vi "create tiff file path.vi"(8 "error in (no error)":errorcluster, 9 "dcimg name":string, 10 "cxd folder Path":path) -> (0 "error IO":errorcluster, 2 "tiff file path":path, 3 "tiff folder path":path)   [LabVIEW 2012, in "DAQOrcaFlash.lvclass"]
uses:
  DAQOrcaFlash.lvclass
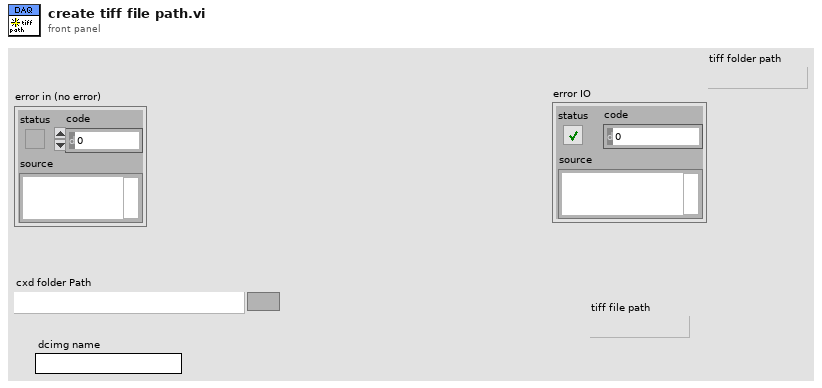
[diagram p1: front panel]
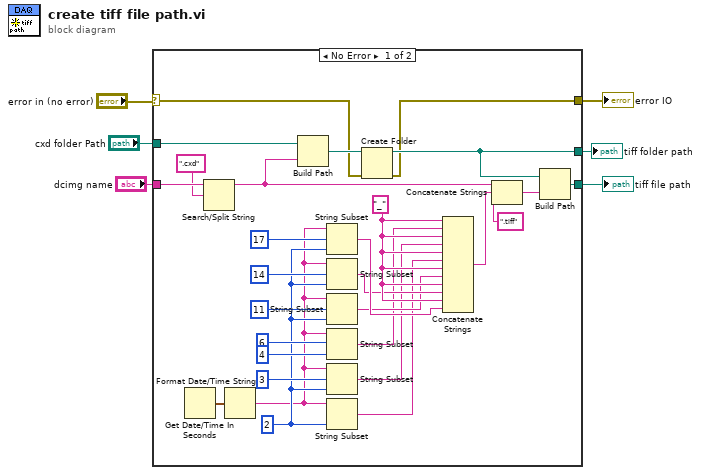
[diagram p0: block diagram]
diagram:
  n1 = case shown="No Error" "error in (no error)" {
    selector: "error in (no error)" -> [w8 w35]
    tunnel: "dcimg name" -> [w16 _]
    tunnel: [w7 w35] -> w4
    tunnel: [w11 _] -> w3
    tunnel: "cxd folder Path" -> [w10 _]
    tunnel: [w9 _] -> w1
    frame No Error {
      w34 = "_" ("string")
      w21 = 2 ("length (rest)")
      n2 = Get Date/Time In Seconds() -> (seconds since 1Jan1904=w19:timestamp)
      n3 = Search/Split String(string=w16, search string/char (-)=".cxd") -> (substring before match=w13:string)  [unwired: 1 in, 2 out]
      n4 = Format Date/Time String(seconds (now)=w19) -> (date/time string=w20:string)  [unwired: 2 in]
      n5 = Build Path(base path=w10, name or relative path=w13) -> (appended path=w14:path)
      n6 = String Subset(string=w20, offset (0)=17, length (rest)=w21) -> (substring=w33:string)
      n7 = String Subset(string=w20, offset (0)=14, length (rest)=w21) -> (substring=w32:string)
      n8 = String Subset(string=w20, offset (0)=11, length (rest)=w21) -> (substring=w31:string)
      n9 = String Subset(string=w20, offset (0)=6, length (rest)=4 ("length (rest)")) -> (substring=w28:string)
      n10 = String Subset(string=w20, offset (0)=3, length (rest)=w21) -> (substring=w29:string)
      n11 = String Subset(string=w20, length (rest)=w21) -> (substring=w30:string)  [unwired: 1 in]
      n12 = Create Folder(path (use dialog)=w14, error in=w8) -> (created path=w9:path, error out=w7:errorcluster)  [unwired: 1 in, 1 out]
      n13 = Concatenate Strings(w34, w28, w34, w29, w34, w30, w34, w31, w34, w32, w34, w33) -> (w18:string)
      n14 = Concatenate Strings(w13, w18, ".tiff" ("string")) -> (w12:string)
      n15 = Build Path(base path=w9, name or relative path=w12) -> (appended path=w11:path)
    }
    frame Error {
    }
  }
  "error IO" <- w4
  "tiff file path" <- w3
  "tiff folder path" <- w1
